vi "Update.vi"(8 "error in (no error)":errorcluster, 11 "Actor in":refnum<class "System Status Actor.lvclass">) -> (0 "error out":errorcluster, 3 "Actor out":refnum<class "System Status Actor.lvclass">)   [LabVIEW 2020, in "System Status Actor.lvclass"]
uses:
  System Status Actor.lvclass
  System Status Actor.lvclass/System Status Actor.ctl
  <vilib>/NI_Real-Time Target Support.lvlib
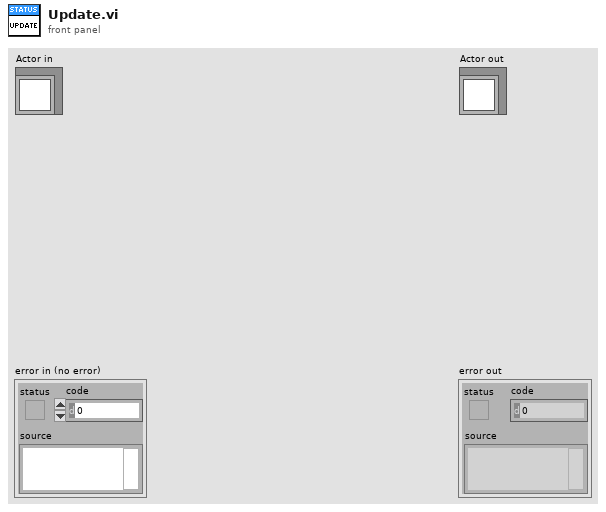
[diagram p1: front panel]
types:
  T1 = typedef "NI_Real-Time Target Support.lvlib/RT CPU Load.ctl" = cluster{"Total (%)":dbl, "Time Critical (%)":dbl, "Timed Structures (%)":dbl, "High (%)":dbl, "Above Normal (%)":dbl, "Normal (%)":dbl, "Background (%)":dbl, "Idle (%)":dbl, "ISR (%)":dbl}
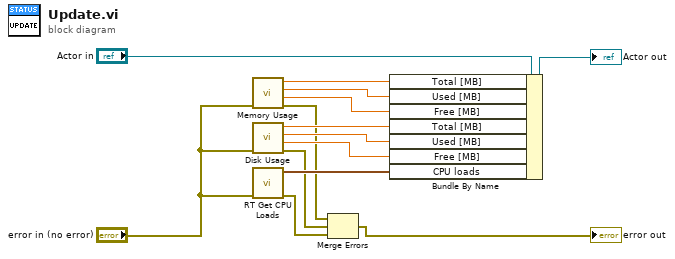
[diagram p0: block diagram]
diagram:
  n1 = call "Memory Usage.vi"("error in (no error)"="error in (no error)") -> ("error out"=w4:errorcluster, "Free [MB]"=w10:dbl, "Used [MB]"=w11:dbl, "Total [MB]"=w12:dbl)  [unwired: 7 in]
  n2 = call "Disk Usage.vi"("error in (no error)"="error in (no error)") -> ("error out"=w3:errorcluster, "Free [MB]"=w7:dbl, "Used [MB]"=w8:dbl, "Total [MB]"=w9:dbl)  [unwired: 7 in]
  n3 = call <vilib>:"RT Get CPU Loads.vi"("error in (no error)"="error in (no error)") -> ("error out"=w2:errorcluster, "CPU loads"=w6:T1[])  [unwired: 9 in]
  n4 = Merge Errors(w4, w3, w2) -> (→"error out":errorcluster)
  n5 = Bundle By Name(cluster="Actor in", "Total [MB]"=w12, "Used [MB]"=w11, "Free [MB]"=w10, "Total [MB]"=w9, "Used [MB]"=w8, "Free [MB]"=w7, "CPU loads"=w6) -> (→"Actor out":refnum<class "System Status Actor.lvclass">)
